vi "Safe Backup Robocopy.vi"(6 "Dest. drive root":path=path "G:/", 7 "Source drive root":path=path "Z:/") -> (0 "Errors out":errorcluster[](array[cluster]), 1 "Commands":string[](array[string]), 3 "End summary":string[](array[string]))   [LabVIEW 2018]
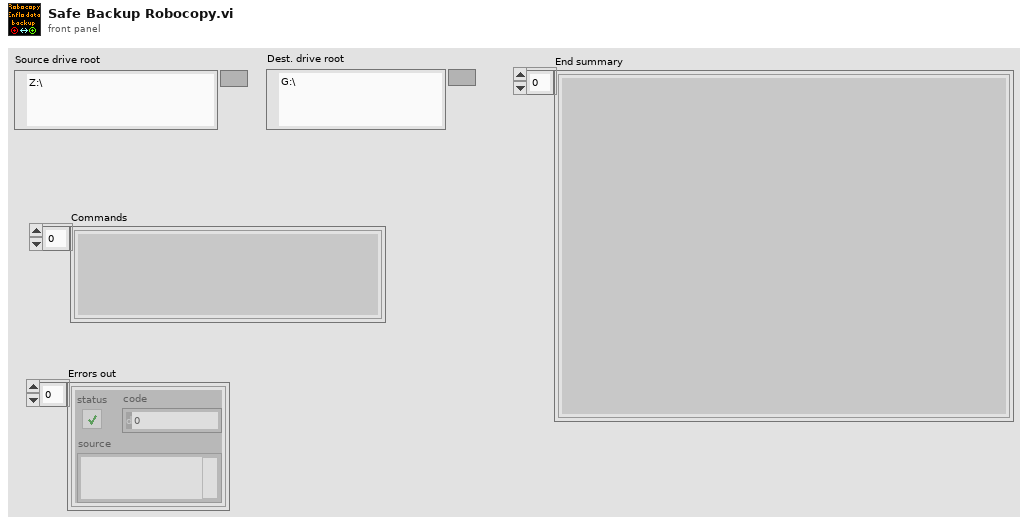
[diagram p1: front panel]
types:
  T1 = enum16{"Zero or one", "One", "Zero or more", "One or more"}
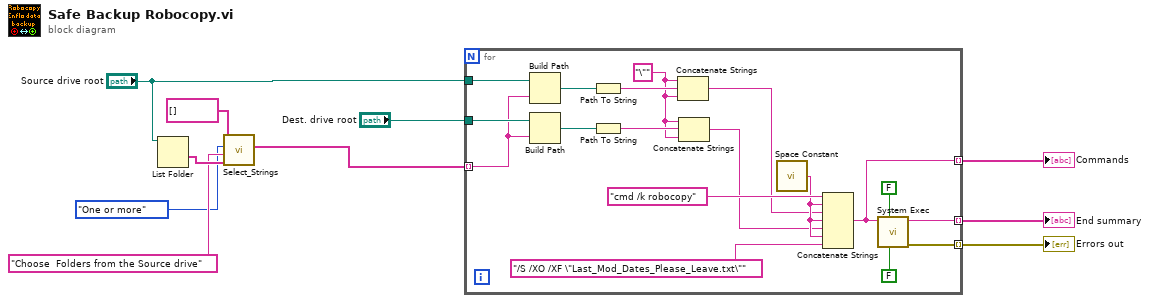
[diagram p0: block diagram]
diagram:
  n1 = List Folder(path="Source drive root") -> (folder names=w5:string[])  [unwired: 3 in, 3 out]
  n2 = call "Select_Strings.vi"("Available Ch names"=w5, "Message"="Choose  Folders from the Source drive", "Selector mode"=T1."One or more", "Desired Ch names (in)"=string[] []) -> ("Selected Channel Names"=w4:string[])  [unwired: 2 in, 2 out]
  n3 = for {
    tunnel: "Source drive root" -> [w26]
    tunnel: "Dest. drive root" -> [w25]
    tunnel: w4 -> [w24] mode=indexing
    tunnel: [w19] -> w9 mode=indexing
    tunnel: [w12] -> w8 mode=indexing
    tunnel: [w11] -> w7 mode=indexing
    w13 = "\"" ("string")
    n4 = Build Path(base path=w26, name or relative path=w24) -> (appended path=w22:path)
    n5 = Build Path(base path=w25, name or relative path=w24) -> (appended path=w21:path)
    n6 = Path To String(path=w22) -> (string=w17:string)
    n7 = Path To String(path=w21) -> (string=w15:string)
    n8 = Concatenate Strings(w13, w17, w13) -> (w16:string)
    n9 = Concatenate Strings(w13, w15, w13) -> (w14:string)
    n10 = call <vilib>:"Space Constant.vi"() -> ("String"=w18:string)
    n11 = Concatenate Strings("cmd /k robocopy", w18, w16, w18, w14, w18, "/S /XO /XF \"Last_Mod_Dates_Please_Leave.txt\"" ("string")) -> (w12:string)
    n12 = call <vilib>:"System Exec.vi"("run minimized? (F)"=FALSE, "wait until completion? (T)"=FALSE, "command line"=w12) -> ("error out"=w19:errorcluster, "standard output"=w11:string)  [unwired: 5 in, 2 out]
  }
  "Errors out" <- w9
  "Commands" <- w8
  "End summary" <- w7
